vi "Begin.vi"(8 "error in":errorcluster) -> (0 "error out":errorcluster)   [LabVIEW 2015]
doc: "Called before other user functions, this VI is expected to open initial I/O refnums, load in file data, and do all program initialization. Notice that the <B>error out</B> terminal is simply used for data flow. Wiring it to other structures or subVIs ensures that this VI runs first."
uses:
  <vilib>/Rock Robotics/WPI/SafetyOutput/WPI_SafetyOutputConfigMenu.ctl
  <vilib>/Rock Robotics/WPI/DriverStation/WPI_DriverStationRobotMode2.ctl
  <vilib>/Rock Robotics/WPI/Joystick/WPI_JoystickDeviceEnum.ctl
  <vilib>/Rock Robotics/SystemInterfaces/DIO/FPGA_DIOPWMChannel.ctl
  <vilib>/Rock Robotics/SystemInterfaces/i2clib/i2c_bus.ctl
  <vilib>/Rock Robotics/SystemInterfaces/DIO/FPGA_DIOChannel.ctl
  Robot Global Data.vi
  <vilib>/Rock Robotics/Network Tables/NT Write String Array.vi
  <vilib>/Rock Robotics/WPI/MotorControl/WPI_MotorControlOpen Talon.vi
  <vilib>/Rock Robotics/WPI/RobotDrive/WPI_RobotDriveOpen4MotorWithExistingMotors.vi
  <vilib>/Rock Robotics/WPI/Switch/WPI_SwitchOpenLimit.vi
  <vilib>/Rock Robotics/WPI/RobotDrive/WPI_RobotDriveOpen2MotorWithExistingMotors.vi
  <vilib>/Rock Robotics/WPI/Gyro/WPI_GyroAnalogOpen.vi
  <vilib>/Rock Robotics/Network Tables/NT Write String.vi
  <vilib>/Rock Robotics/SystemInterfaces/AI/FPGA_AIGyroChannel.ctl
  <vilib>/Rock Robotics/SystemInterfaces/AI/FPGA_AIChannel.ctl
panel:
  out "BadCal Mag":bool
  out "BadCal Accel":bool
  out "BadCal Gyro":bool
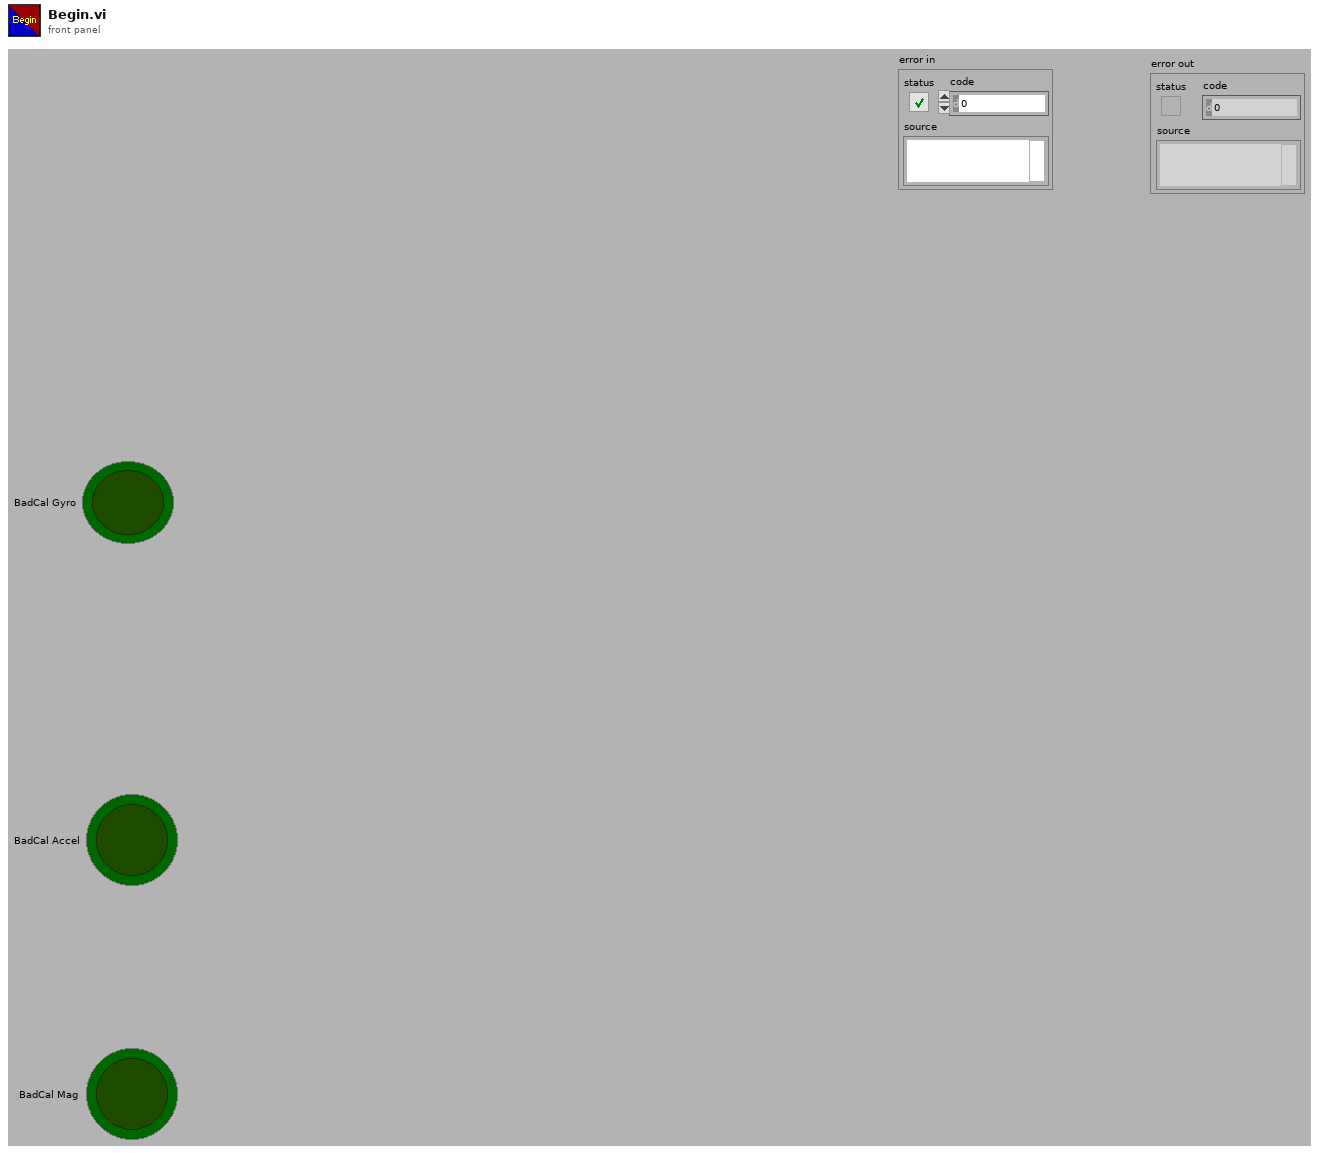
[diagram p1: front panel]
types:
  T1 = typedef "WPI_JoystickDeviceEnum.ctl" = enum16{"USB 0", "USB 1", "USB 2", "USB 3", "USB 4", "USB 5"}
  T2 = typedef "WPI_DriverStationRobotMode2.ctl" = enum16{"Autonomous Disabled", "Autonomous Enabled", "Teleop Disabled", "Teleop Enabled", "Disconnected", "Finish", "Test Disabled", "Test Enabled", "Emergency Stopped"}
  T3 = typedef "WPI_SafetyOutputConfigMenu.ctl" = enum16{"Enable", "Disable"}
  T4 = typedef "FPGA_DIOChannel.ctl" = enum8{"DIO 0", "DIO 1", "DIO 2", "DIO 3", "DIO 4", "DIO 5", "DIO 6", "DIO 7", "DIO 8", "DIO 9", "DIO MXP 0", "DIO MXP 1", "DIO MXP 2", "DIO MXP 3", "DIO MXP 4", "DIO MXP 5", "DIO MXP 6", "DIO MXP 7", "DIO MXP 8", "DIO MXP 9", "DIO MXP 10", "DIO MXP 11", "DIO MXP 12", "DIO MXP 13", "DIO MXP 14", "DIO MXP 15", "Invalid"}
  T5 = typedef "i2c_bus.ctl" = enum16{"I2C On-Board", "I2C MXP", "Invalid"}
  T6 = cluster{"Data Rate":enum8{"0.75 Hz", "1.5 Hz", "3.0 Hz", "7.5 Hz", "15 Hz", "30 Hz", "75 Hz", "220 Hz"}, "Range":u8, "Sense Enable":bool, "Mag Scale":cluster{"Xscale":dbl, "Yscale":dbl, "Zscale":dbl}, "Mag Offset":cluster{"Xzero":dbl, "Yzero":dbl, "Zzero":dbl}, "Anomaly Thresh":dbl, "Local Mag":dbl}
  T7 = cluster{"Data Rate":enum8{"100 Hz", "200 Hz", "400 Hz", "800 Hz"}, "Range":u8, "HPF Enable":bool, "HPCF":enum8{"0000", "0001", "0010", "0011", "0100", "0101", "0110", "0111", "1000", "1001"}, "Sense Enable":bool}
  T8 = cluster{"Data Rate":enum8{"Power-down mode", "1 Hz", "10 Hz", "25 Hz", "50 Hz", "100 Hz", "200 Hz", "400 Hz", "Low-power mode only", "1.344 kHz"}, "Range":u8, "HPF Enable":bool, "HPCF":enum8{"00", "01", "10", "11"}, "Sense Enable":bool, "Accel Scale":cluster{"Xscale":dbl, "Yscale":dbl, "Zscale":dbl}, "Motion Thresh":dbl}
  T9 = typedef "FPGA_DIOPWMChannel.ctl" = enum8{"PWM 0", "PWM 1", "PWM 2", "PWM 3", "PWM 4", "PWM 5", "PWM 6", "PWM 7", "PWM 8", "PWM 9", "PWM MXP 0", "PWM MXP 1", "PWM MXP 2", "PWM MXP 3", "PWM MXP 4", "PWM MXP 5", "PWM MXP 6", "PWM MXP 7", "PWM MXP 8", "PWM MXP 9", "Invalid"}
  T10 = typedef "FPGA_AIChannel.ctl" = enum8{"AI 0", "AI 1", "AI 2", "AI 3", "AI MXP 0", "AI MXP 1", "AI MXP 2", "AI MXP 3", "Invalid"}
  T11 = typedef "FPGA_AIGyroChannel.ctl" = enum8{"AI 0", "AI 1", "Invalid"}
  T12 = typedef "WPI_SwitchDevRef.ctl" = cluster{"DevStatus":errorcluster, "DIO Channel":T4, "CntIndex":T13, "Normally Closed":bool}
  T13 = typedef "FPGA_CounterCtrSystemIndex.ctl" = enum8{"Ctr 0", "Ctr 1", "Ctr 2", "Ctr 3", "Ctr 4", "Ctr 5", "Ctr 6", "Ctr 7", "Invalid"}
  T14 = typedef "WPI_PotentiometerDevRef.ctl" = cluster{"DevStatus":errorcluster, "Analog Channel":T10, "Invert Output":bool}
  T15 = cluster{"BadCal Gyro":bool, "BadCal Accel":bool, "BadCal Mag":bool}
  T16 = typedef "IMUDevRef.ctl" = cluster{"DevStatus":errorcluster, "Gyro Address":u8, "Gyro Range":u8, "Mean Rates":cluster{"Xmo":dbl, "Ymo":dbl, "Zmo":dbl}, "StdDev Rates":cluster{"Xsdo":dbl, "Ysdo":dbl, "Zsdo":dbl}, "Fast":bool, "Reset":bool, "Accel Address":u8, "Accel Range":u8, "Accel Scale":cluster{"Xscale":dbl, "Yscale":dbl, "Zscale":dbl}, "Mag Address":u8, "Mag Range":u8, "G Sense":bool, "A Sense":bool, "M Sense":bool, "Accel Offset":cluster{"Xzero":dbl, "Yzero":dbl, "Zzero":dbl}, "Motion Thresh":dbl, "Mag Scale":cluster{"Xscale":dbl, "Yscale":dbl, "Zscale":dbl}, "Mag Offset":cluster{"Xzero":dbl, "Yzero":dbl, "Zzero":dbl}, "I2C Bus":T5, "Handle":i32, "Anomaly Thresh":dbl, "Local Mag":dbl}
  T17 = typedef "WPI_MotorControlDeviceRef.ctl" = cluster{"DeviceStatus":errorcluster, "Type":T18, "PWM":cluster{"PWM Channel":T9, "DeadBand":T19}, "CAN":cluster{"Device Number":u8, "Control Mode":T20, "Semaphore":T21, "Max Vout":dbl, "TalonSRX Control Mode":T22}, "Invert":bool}
  T18 = typedef "WPI_MotorControlType.ctl" = enum16{"PWM", "CAN", "CANTalonSRX"}
  T19 = typedef "WPI_PWMDeadband.ctl" = cluster{"Name":string, "maxPositivePwm":i32, "minPositivePwm":i32, "centerPwm":i32, "maxNegativePwm":i32, "minNegativePwm":i32, "angularRange":u16}
  T20 = typedef "WPI_CANJaguar_ControlMode.ctl" = enum8{"Percent VBus", "Current", "Speed", "Position", "Voltage"}
  T21 = typedef "Semaphore RefNum" = refnum<k1>
  T22 = typedef "WPI_CANTalonSRX_APIControlMode.ctl" = enum8{"Percent VBus", "Speed", "Position", "Slave", "Unchanged / Invalid", "Voltage Compensation", "Current", "Motion Profile"}
  T23 = typedef "WPI_DigitalInputDevRef.ctl" = cluster{"DevStatus":errorcluster, "DIO Channel":T4}
  T24 = typedef "WPI_RobotDriveDevRef.ctl" = cluster{"DevStatus":errorcluster, "Motors[]":T17[], "Square Inputs":bool, "Max Output":dbl}
  T25 = typedef "WPI_GyroDevRef.ctl" = cluster{"DevStatus":errorcluster, "Analog Channel":T10, "Offset":dbl, "Gain (VoltsPerDegree/Second)":dbl, "Gyro Type":enum16{"Analog", "XRS450"}, "Handle":i32, "SPI Bus":T26, "Device Found":bool, "Sample Rate":dbl, "Calibrate On Open":bool}
  T26 = typedef "spi_bus.ctl" = enum16{"SPI On-Board, CS0", "SPI On-Board, CS1", "SPI On-Board, CS2", "SPI On-Board, CS3", "SPI MXP", "Invalid"}
  T27 = typedef "WPI_JoystickDevRef.ctl" = cluster{"Device":T1}
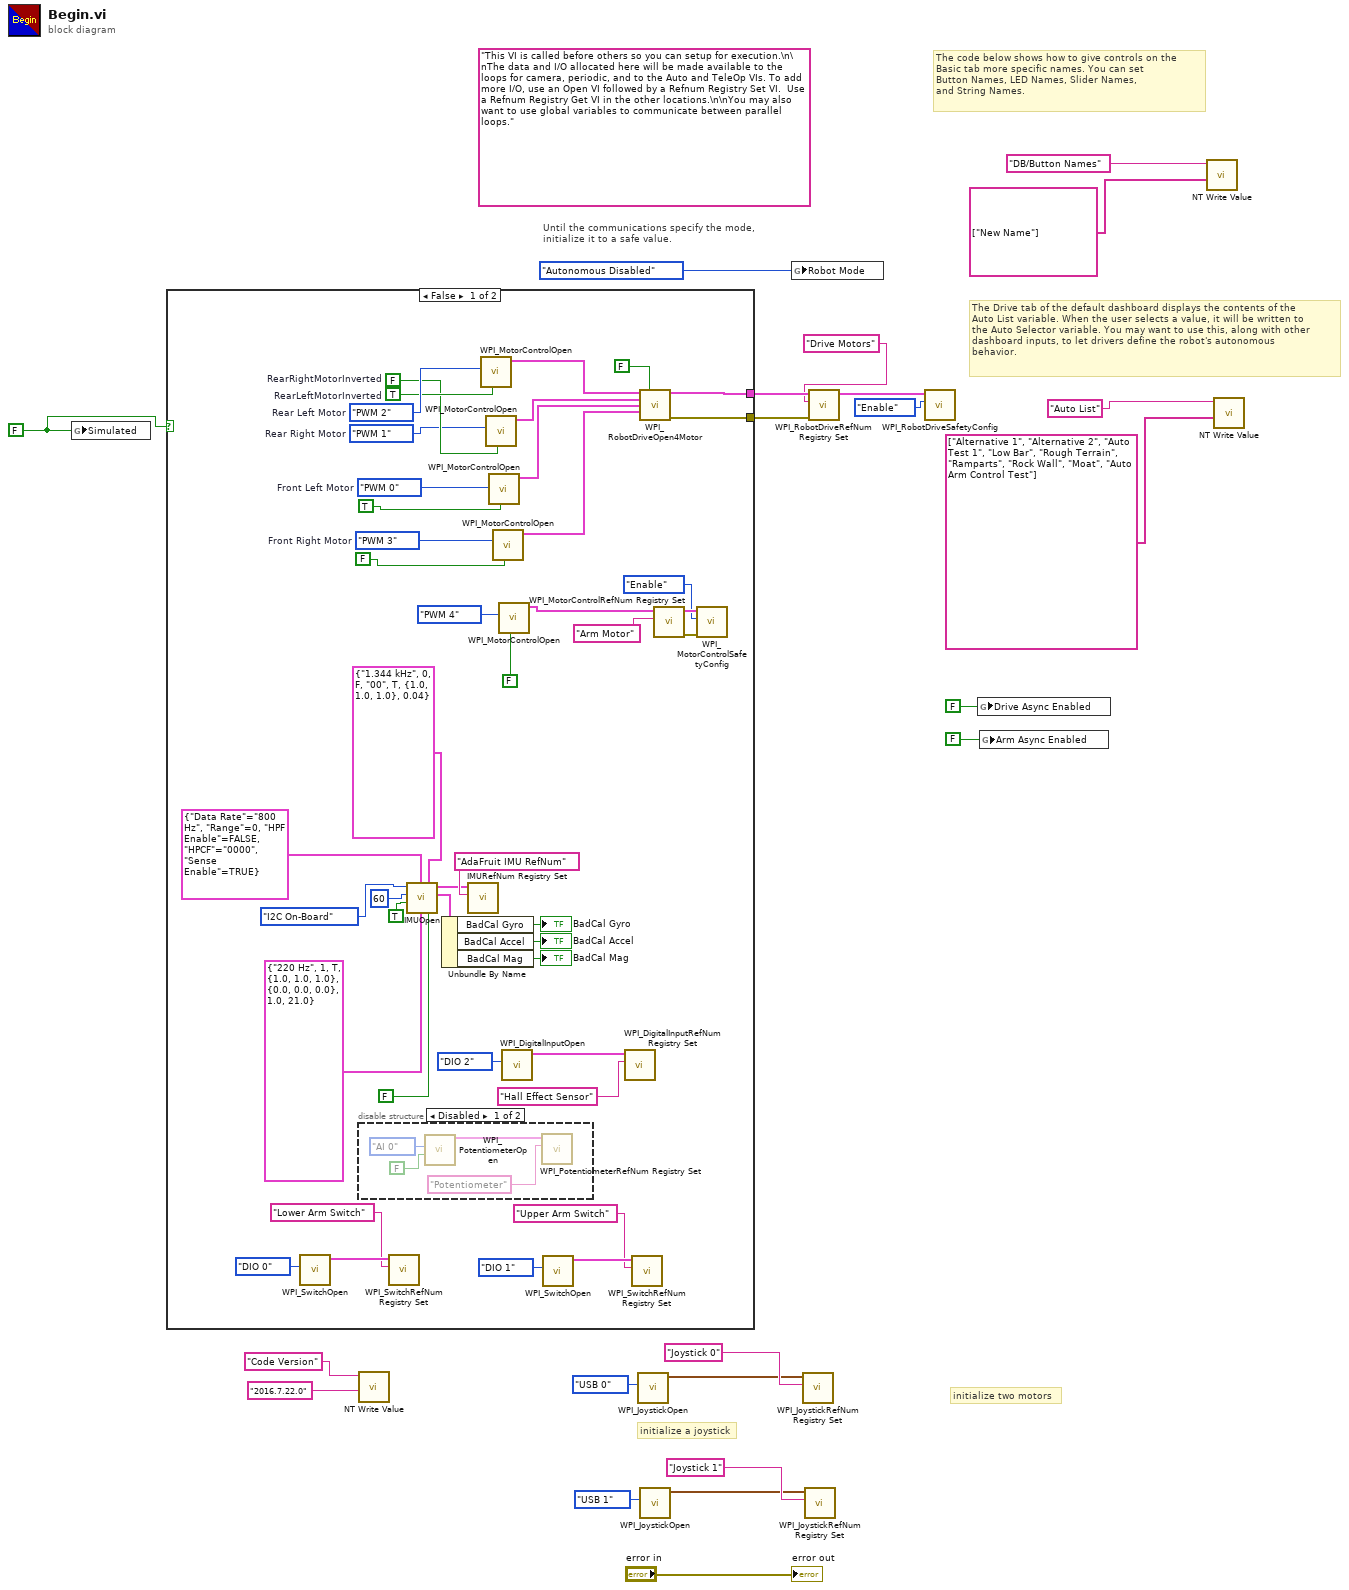
[diagram p0: block diagram]
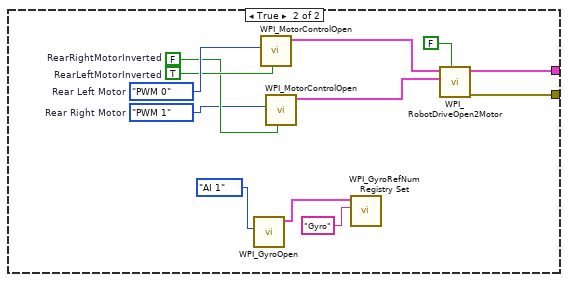
[diagram p3: hidden frame]
diagram:
  w5 = FALSE ("Simulated")
  (unwired) "This VI is called before others so you can setup for execution.\n\nThe data and I/O allocated here will be made available to the loops for camera, periodic, and to the Auto and TeleOp VIs. To add more I/O, use an Open VI followed by a Refnum Registry Set VI.  Use a Refnum Registry Get VI in the other locations.\n\nYou may also want to use global variables to communicate between parallel loops."
  # "The Drive tab of the default dashboard displays the contents of the\nAuto List variable. When the user selects a value, it will be written to\nthe Auto Selector variable. You may want to use this, along with other\ndashboard inputs, to let drivers define the robot's autonomous\nbehavior."
  # "The code below shows how to give controls on the\nBasic tab more specific names. You can set\nButton Names, LED Names, Slider Names,\nand String Names."
  # "initialize a joystick"
  # "Until the communications specify the mode,\ninitialize it to a safe value."
  # "initialize two motors"
  n1 = global write "Robot Global Data.vi" "Simulated"(w5) -> ()
  n2 = case shown="False" w5 {
    tunnel: [w66 w82] -> w22
    tunnel: [w65 w81] -> w20
    frame False {
      w60 = FPGA_DIOPWMChannel."PWM 3"  # Front Right Motor
      w58 = FPGA_DIOPWMChannel."PWM 0"  # Front Left Motor
      w53 = FPGA_DIOPWMChannel."PWM 1"  # Rear Right Motor
      w56 = FPGA_DIOPWMChannel."PWM 2"  # Rear Left Motor
      w55 = TRUE  # RearLeftMotorInverted
      w54 = FALSE  # RearRightMotorInverted
      n3 = call-poly <vilib>:"WPI_SwitchOpen.vi"("DIO Channel"=FPGA_DIOChannel."DIO 0") -> ("SwitchDevRef"=w32:T12)  [unwired: 9 in, 1 out]
      n4 = disable-structure shown="Disabled" {
        frame Disabled {
          n5 = call <vilib>:"WPI_PotentiometerOpen.vi"("Invert Output"=FALSE, "Analog Channel"=FPGA_AIChannel."AI 0") -> ("PotDevRef"=w67:T14)  [unwired: 8 in, 1 out]
          n6 = call <vilib>:"WPI_PotentiometerRefNum Registry Set.vi"("refnum name"="Potentiometer", "PotDevRef"=w67) -> ()  [unwired: 8 in, 2 out]
        }
        frame Enabled {
        }
      }
      n7 = call <vilib>:"WPI_SwitchRefNum Registry Set.vi"("refnum name"="Lower Arm Switch", "SwitchDevRef"=w32) -> ()  [unwired: 8 in, 2 out]
      n8 = call "IMUOpen.vi"("MagCal"=FALSE, "Accel Set"=T8 {"Data Rate"=enum."1.344 kHz", "Range"=0, "HPF Enable"=FALSE, "HPCF"=enum."00", "Sense Enable"=TRUE, "Accel Scale"={"Xscale"=1.0, "Yscale"=1.0, "Zscale"=1.0}, "Motion Thresh"=0.04}, "Mag Set"=T6 {"Data Rate"=enum."220 Hz", "Range"=1, "Sense Enable"=TRUE, "Mag Scale"={"Xscale"=1.0, "Yscale"=1.0, "Zscale"=1.0}, "Mag Offset"={"Xzero"=0.0, "Yzero"=0.0, "Zzero"=0.0}, "Anomaly Thresh"=1.0, "Local Mag"=21.0}, "Gyro Set"=T7 {"Data Rate"=enum."800 Hz", "Range"=0, "HPF Enable"=FALSE, "HPCF"=enum."0000", "Sense Enable"=TRUE}, "Fast"=TRUE, "CalSamples"=60 ("CalAvg"), "I2C Bus"=i2c_bus."I2C On-Board") -> ("Cal Result"=w37:T15, "AdaIMUDevRef Out"=w35:T16)  [unwired: 2 in, 1 out]
      n9 = Unbundle By Name(w37) -> ("BadCal Gyro"=→"BadCal Gyro":bool, "BadCal Accel"=→"BadCal Accel":bool, "BadCal Mag"=→"BadCal Mag":bool)
      n10 = call "IMURefNum Registry Set.vi"("refnum name"="AdaFruit IMU RefNum", "AdaIMUDevRef"=w35) -> ()  [unwired: 8 in, 2 out]
      n11 = call-poly <vilib>:"WPI_MotorControlOpen.vi"("Invert"=w55, "PWM Channel"=w56) -> ("MotorControlDeviceRef"=w64:T17)  [unwired: 8 in, 1 out]
      n12 = call-poly <vilib>:"WPI_MotorControlOpen.vi"("Invert"=w54, "PWM Channel"=w53) -> ("MotorControlDeviceRef"=w63:T17)  [unwired: 8 in, 1 out]
      n13 = call-poly <vilib>:"WPI_MotorControlOpen.vi"("Invert"=TRUE ("Front Left Motor Inverted"), "PWM Channel"=w58) -> ("MotorControlDeviceRef"=w62:T17)  [unwired: 8 in, 1 out]
      n14 = call-poly <vilib>:"WPI_MotorControlOpen.vi"("Invert"=FALSE ("Front Right Motor Inverted"), "PWM Channel"=w60) -> ("MotorControlDeviceRef"=w61:T17)  [unwired: 8 in, 1 out]
      n15 = call-poly <vilib>:"WPI_MotorControlOpen.vi"("Invert"=FALSE, "PWM Channel"=FPGA_DIOPWMChannel."PWM 4") -> ("MotorControlDeviceRef"=w51:T17)  [unwired: 8 in, 1 out]
      n16 = call <vilib>:"WPI_DigitalInputOpen.vi"("DIO Channel"=FPGA_DIOChannel."DIO 2") -> ("DigitalInputDevRef"=w25:T23)  [unwired: 9 in, 1 out]
      n17 = call-poly <vilib>:"WPI_SwitchOpen.vi"("DIO Channel"=FPGA_DIOChannel."DIO 1") -> ("SwitchDevRef"=w29:T12)  [unwired: 9 in, 1 out]
      n18 = call <vilib>:"WPI_DigitalInputRefNum Registry Set.vi"("refnum name"="Hall Effect Sensor", "DigitalInputDevRef"=w25) -> ()  [unwired: 8 in, 2 out]
      n19 = call <vilib>:"WPI_SwitchRefNum Registry Set.vi"("refnum name"="Upper Arm Switch", "SwitchDevRef"=w29) -> ()  [unwired: 8 in, 2 out]
      n20 = call-poly <vilib>:"WPI_RobotDriveOpen4Motor.vi"("Rear Left Motor Dev Ref"=w64, "Square Inputs"=FALSE, "Rear Right Motor Dev Ref"=w63, "Front Left Motor Dev Ref"=w62, "Front Right Motor Dev Ref"=w61) -> ("RobotDriveDevRef"=w66:T24, "error out"=w65:errorcluster)  [unwired: 9 in]
      n21 = call <vilib>:"WPI_MotorControlRefNum Registry Set.vi"("refnum name"="Arm Motor", "MotorControlDevRef"=w51) -> ("error out"=w48:errorcluster, "MotorControlDevRef"=w47:T17)  [unwired: 8 in]
      n22 = call <vilib>:"WPI_MotorControlSafetyConfig.vi"("error in (no error)"=w48, "mode"=WPI_SafetyOutputConfigMenu."Enable", "MotorControlDevRef"=w47) -> ()  [unwired: 7 in, 2 out]
    }
    frame True {
      w77 = FPGA_DIOPWMChannel."PWM 1"  # Rear Right Motor
      w80 = FPGA_DIOPWMChannel."PWM 0"  # Rear Left Motor
      w79 = TRUE  # RearLeftMotorInverted
      w78 = FALSE  # RearRightMotorInverted
      n23 = call-poly <vilib>:"WPI_GyroOpen.vi"("Analog Channel"=FPGA_AIGyroChannel."AI 1") -> ("GyroDevRef"=w71:T25)  [unwired: 8 in, 2 out]
      n24 = call-poly <vilib>:"WPI_MotorControlOpen.vi"("Invert"=w79, "PWM Channel"=w80) -> ("MotorControlDeviceRef"=w75:T17)  [unwired: 8 in, 1 out]
      n25 = call-poly <vilib>:"WPI_MotorControlOpen.vi"("Invert"=w78, "PWM Channel"=w77) -> ("MotorControlDeviceRef"=w74:T17)  [unwired: 8 in, 1 out]
      n26 = call <vilib>:"WPI_GyroRefNum Registry Set.vi"("refnum name"="Gyro", "GyroDevRef"=w71) -> ()  [unwired: 8 in, 2 out]
      n27 = call-poly <vilib>:"WPI_RobotDriveOpen2Motor.vi"("Square Inputs"=FALSE, "Right Motor Dev Ref"=w74, "Left Motor Dev Ref"=w75) -> ("error out"=w81:errorcluster, "RobotDriveDevRef"=w82:T24)  [unwired: 7 in]
    }
  }
  n28 = call-poly <vilib>:"NT Write Value.vi"("String"="2016.7.22.0", "Name"="Code Version") -> ()  [unwired: 9 in, 1 out]
  n29 = call <vilib>:"WPI_JoystickOpen.vi"("JoystickDevice"=WPI_JoystickDeviceEnum."USB 0") -> ("JoystickDevRef"=w15:T27)  [unwired: 10 in]
  n30 = call <vilib>:"WPI_JoystickOpen.vi"("JoystickDevice"=WPI_JoystickDeviceEnum."USB 1") -> ("JoystickDevRef"=w7:T27)  [unwired: 10 in]
  n31 = global write "Robot Global Data.vi" "Robot Mode"(WPI_DriverStationRobotMode2."Autonomous Disabled" ("Robot Mode")) -> ()
  n32 = call <vilib>:"WPI_JoystickRefNum Registry Set.vi"("refnum name"="Joystick 0", "JoystickDevRef"=w15) -> ()  [unwired: 8 in, 2 out]
  n33 = call <vilib>:"WPI_JoystickRefNum Registry Set.vi"("refnum name"="Joystick 1", "JoystickDevRef"=w7) -> ()  [unwired: 8 in, 2 out]
  n34 = call <vilib>:"WPI_RobotDriveRefNum Registry Set.vi"("error in (no error)"=w20, "refnum name"="Drive Motors", "RobotDriveDevRef"=w22) -> ("RobotDriveDevRef"=w19:T24)  [unwired: 1 in, 7 out]
  n35 = call <vilib>:"WPI_RobotDriveSafetyConfig.vi"("mode"=WPI_SafetyOutputConfigMenu."Enable", "RobotDriveDevRef"=w19) -> ()  [unwired: 8 in, 2 out]
  n36 = global write "Robot Global Data.vi" "Drive Async Enabled"(FALSE ("Drive Async")) -> ()
  n37 = global write "Robot Global Data.vi" "Arm Async Enabled"(FALSE ("Drive Async")) -> ()
  n38 = call-poly <vilib>:"NT Write Value.vi"("String Array"=string[] ["New Name"], "Name"="DB/Button Names") -> ()  [unwired: 9 in, 1 out]
  n39 = call-poly <vilib>:"NT Write Value.vi"("String Array"=string[] ["Alternative 1", "Alternative 2", "Auto Test 1", "Low Bar", "Rough Terrain", "Ramparts", "Rock Wall", "Moat", "Auto Arm Control Test"], "Name"="Auto List") -> ()  [unwired: 9 in, 1 out]
  "error out" <- "error in"
